vi "InsertPanelToMainframe.vi"(8 "error in (no error)":errorcluster, 9 "VI Refnum":refnum<vi>, 10 "Sub Panel":string, 11 "MicroscopeControllerIO in":refnum<class "MicroscopeControllerIO.lvclass">) -> (0 "error out":errorcluster, 3 "MicroscopeControllerIO out":refnum<class "MicroscopeControllerIO.lvclass">)   [LabVIEW 2020, in "MicroscopeControllerIO.lvclass"]
uses:
  MicroscopeControllerIO.lvclass
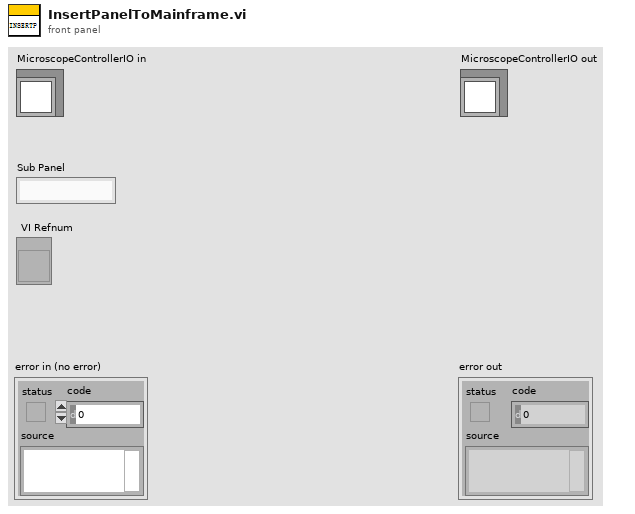
[diagram p1: front panel]
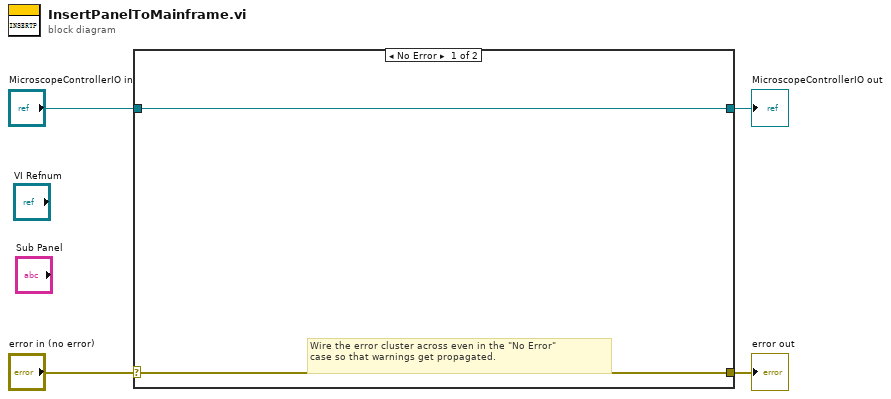
[diagram p0: block diagram]
diagram:
  n1 = case shown="No Error" "error in (no error)" {
    selector: "error in (no error)" -> [w5 w8]
    tunnel: [w5 w8] -> w3
    tunnel: [w6 w7] -> w1
    tunnel: "MicroscopeControllerIO in" -> [w6 w7]
    frame No Error {
      # "Wire the error cluster across even in the \"No Error\"\ncase so that warnings get propagated."
    }
    frame Error {
    }
  }
  "error out" <- w3
  "MicroscopeControllerIO out" <- w1
